vi "RSZVB Set TRM Power Amplifier State.vi"(7 "Power Amplifier State (Off)":bool, 8 "error in (no error)":errorcluster {"code" format="%.0x"}, 9 "Path (1)":i32=1, 10 "Channel (1)":i32=1, 11 "VISA resource name":refnum<visa-resource-name>) -> (0 "error out":errorcluster {"code" format="%.0x"}, 3 "VISA resource name out":refnum<visa-resource-name>)   [LabVIEW 2011]
doc: "This VI loops an internal power amplifier into one of the RF signal paths (source paths).\n\nRemote-control command(s):\n[SENSe<Ch>:]TEUNit:PAMPlifier<Path>[:STATe]"
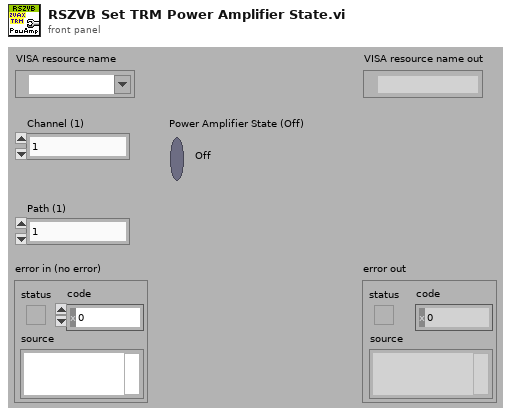
[diagram p1: front panel]
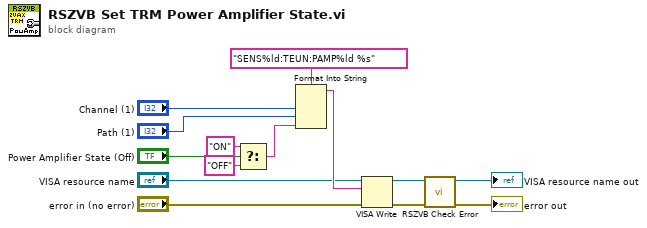
[diagram p0: block diagram]
diagram:
  n1 = Select(t="ON", s="Power Amplifier State (Off)", f="OFF") -> (s? t:f=w10:string)
  n2 = Format Into String(format string="SENS%ld:TEUN:PAMP%ld %s", "Channel (1)", "Path (1)", w10) -> (resulting string=w9:string)  [unwired: 2 in, 1 out]
  n3 = VISA Write(VISA resource name="VISA resource name", write buffer=w9, error in (no error)="error in (no error)") -> (VISA resource name out=w13:refnum<visa-resource-name>, error out=w14:errorcluster)  [unwired: 1 out]
  n4 = call "RSZVB Check Error.vi"("error in (no error)"=w14, "VISA session"=w13) -> ("error out"=→"error out":errorcluster, "dup VISA session"=→"VISA resource name out":refnum<visa-resource-name>)  [unwired: 8 in]
